vi "Initialize.vi"(8 "error in (no error)":errorcluster, 10 "Simulated Custom Devices":refnum<class "Simulated VeriStand Custom Device.lvclass">[](array[class]), 11 "Simulated VeriStand Engine in":refnum<class "Simulated VeriStand Engine.lvclass">) -> (0 "error out":errorcluster, 3 "Simulated VeriStand Engine out":refnum<class "Simulated VeriStand Engine.lvclass">)   [LabVIEW 2016, in "Simulated VeriStand Engine.lvclass"]
uses:
  Simulated VeriStand Engine.lvclass
  Simulated VeriStand Custom Device/Simulated VeriStand Custom Device.lvclass
  Simulated VeriStand Engine.lvclass/Simulated VeriStand Engine.ctl
  <vilib>/NI Veristand/Custom Device API/Data Table Ref.ctl
  Typedefs/DSF.Engine.Pointers.Control.ctl
  Source/Submodules/Memory/Source/Classes/Internal/Memory.Pointer.Internal.lvclass
  C:/Git/SourceTree/DSF/Source/Submodules/Memory/Source/Classes/Pointer/Memory.Pointer.lvclass
  Typedefs/DSF.Engine.Pointers.Status.ctl
  Source/Submodules/Memory/Source/Classes/Pointer/Memory.Pointer.lvclass/Memory.Pointer.ctl
  Source/Submodules/Memory/Source/Classes/Pointer/Memory.Pointer.Write.Safe.0D.Bool.vi
  Source/Submodules/Memory/Source/Classes/Pointer/Memory.Pointer.Write.Safe.0D.U32.vi
  Source/Submodules/Memory/Source/Classes/Pointer/Memory.Pointer.Write.Unsafe.0D.Bool.vi
  Source/Submodules/Memory/Source/Classes/Pointer/Memory.Pointer.Parameter Check.Null Pointer.vi
  Source/Submodules/Memory/Source/Classes/Pointer/Memory.Pointer.Parameter Check.Subset.vi
  Source/Submodules/Memory/Source/Classes/Pointer/Memory.Pointer.Write.Unsafe.0D.U32.vi
  Source/Submodules/Memory/Source/Classes/Pointer/Memory.Pointer.Get Address.vi
  Source/Submodules/Memory/Source/Classes/Pointer/Memory.Pointer.Errors.vi
  Source/Submodules/Memory/Source/Classes/Pointer/Memory.Pointer.Errors.Null Pointer.vi
  Source/Submodules/Memory/Source/Classes/Pointer/Memory.Pointer.Errors.Out of Bounds.vi
  Source/Submodules/Memory/Source/Classes/Pointer/Memory.Pointer.Get Size.vi
  Source/Submodules/Memory/Source/Classes/Pointer/Memory.Pointer.Errors.Create Error.vi
  Source/Submodules/Memory/Source/Submodules/SEH/Source/VIs/Static Error Handling.Source Buffer.Write.String.vi
  Source/Submodules/Memory/Source/Classes/Pointer/Memory.Pointer.Errors.Write Pointer Size.vi
  Source/Submodules/Memory/Source/Submodules/SEH/Source/VIs/Static Error Handling.Source Buffer.Write.Numeric.Scalar.Base10.vi
  Source/Submodules/Memory/Source/Submodules/SEH/Source/VIs/Static Error Handling.Source Buffer.Write.Numeric.Scalar.Base10 (U64).vi
  Source/Submodules/Memory/Source/Submodules/SEH/Source/VIs/Static Error Handling.Error Cluster Constant.vi
  Source/Submodules/Memory/Source/Submodules/SEH/Source/VIs/Static Error Handling.Error Cluster Constant (256B).vi
  Source/Submodules/Memory/Source/Submodules/SEH/Source/VIs/Static Error Handling.Parameters.Status.Set.vi
  Source/Submodules/Memory/Source/Submodules/SEH/Source/VIs/Static Error Handling.Parameters.Code.Set.vi
  Source/Submodules/Memory/Source/Submodules/SEH/Source/VIs/Static Error Handling.Parameters.VI Source.Set.vi
  Source/Submodules/Memory/Source/Constants/Memory.Constants.vi
  Source/Submodules/Memory/Source/Constants/Memory.Constants.Library Name.vi
  Source/Submodules/Memory/Source/Classes/Pointer/Memory.Pointer.Errors.Get Info.vi
  Source/Submodules/Memory/Source/Classes/Internal/Memory.Pointer.Internal.Allocate.vi
  <vilib>/NI Veristand/Custom Device API/Global Data Refs.vi
  <vilib>/NI Veristand/Custom Device API/Custom Device API.lvlib
  Source/Submodules/Memory/Source/Classes/Pointer/Memory.Pointer.lvclass
panel:
  in  "Channel Count":u32
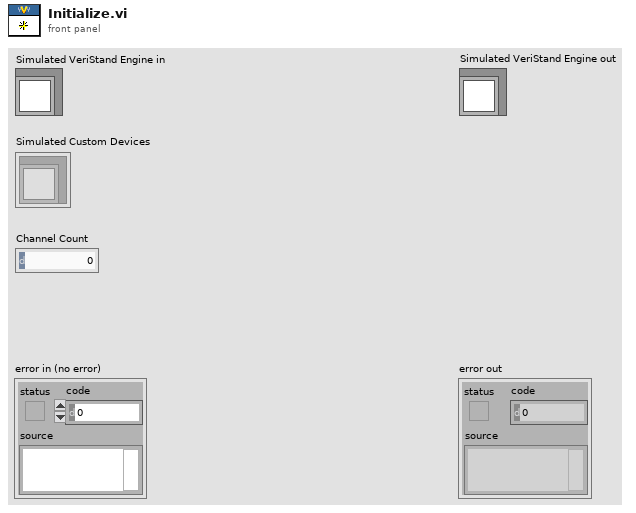
[diagram p1: front panel]
types:
  T1 = typedef "Simulated VeriStand Engine.lvclass/DSF.Engine.Pointers.Status.ctl" = cluster{"actual period":refnum<class "Memory.Pointer.Internal.lvclass">}
  T2 = typedef "Simulated VeriStand Engine.lvclass/DSF.Engine.Pointers.Control.ctl" = cluster{"stop":refnum<class "Memory.Pointer.Internal.lvclass">, "target period":refnum<class "Memory.Pointer.Internal.lvclass">}
  T3 = typedef "Custom Device API.lvlib/Data Table Ref.ctl" = cluster{"Ptr.Beg":u64, "Ptr.End":u64}
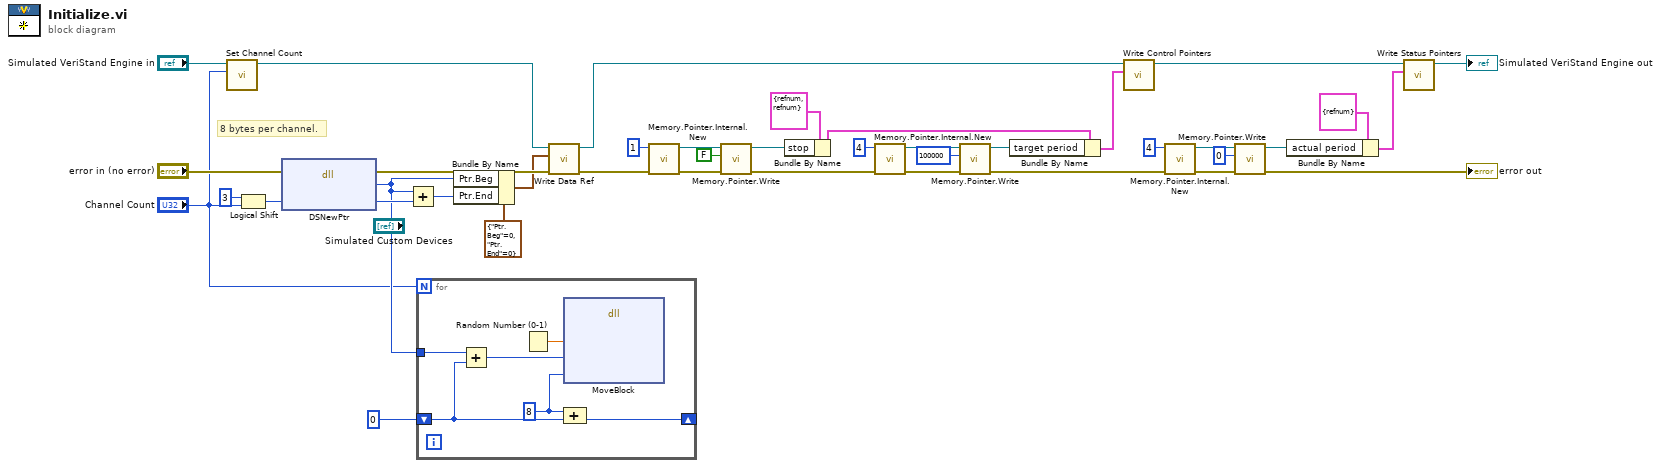
[diagram p0: block diagram]
diagram:
  # "8 bytes per channel."
  n1 = call "Set Channel Count.vi"("Channel Count"="Channel Count", "Simulated VeriStand Engine in"="Simulated VeriStand Engine in") -> ("Simulated VeriStand Engine out"=w2:refnum<class "Simulated VeriStand Engine.lvclass">)  [unwired: 8 in, 1 out]
  n2 = Logical Shift(y=i16 3, x="Channel Count") -> (x << y=w39:u32)
  n3 = dll-call lib="LabVIEW" fn="DSNewPtr"(error in="error in (no error)", "size"=w39) -> (error out=w5:errorcluster, "pointer"=w8:u64, "size"=w36:u32)  [unwired: 2 in, 1 out]
  n4 = Add(x=w8, y=w36) -> (x+y=w37:u64)
  n5 = for {
    N: "Channel Count" -> [_]
    tunnel: w8 -> [w45]
    shift-right: [w44] -> _
    shift-left: u64 0 -> [w43]
    w41 = u64 8
    n6 = Add(x=w45, y=w43) -> (x+y=w42:u64)
    n7 = Random Number (0-1)() -> (number: 0 to 1=w46:dbl)
    n8 = dll-call lib="LabVIEW" fn="MoveBlock"("src"=w46, "dst"=w42, "size"=w41) -> ()  [unwired: 7 in, 2 out]
    n9 = Compound Arithmetic op=ADD(w41, w43) -> (w44:u64)
  }
  n10 = Bundle By Name(cluster=T3 {"Ptr.Beg"=0, "Ptr.End"=0} ("Data Ref"), "Ptr.Beg"=w8, "Ptr.End"=w37) -> (w3:T3)
  n11 = call "Write Data Ref.vi"("error in (no error)"=w5, "Data Table Ref"=w3, "Simulated VeriStand Engine in"=w2) -> ("error out"=w4:errorcluster, "Simulated VeriStand Engine out"=w1:refnum<class "Simulated VeriStand Engine.lvclass">)  [unwired: 7 in]
  n12 = call "Memory.Pointer.Internal.New.vi"("error in (no error)"=w4, "size"=u64 1) -> ("error out"=w22:errorcluster, "pointer"=w23:refnum<class "Memory.Pointer.Internal.lvclass">)  [unwired: 8 in]
  n13 = call-poly "Memory.Pointer.Write.vi"("error in (no error)"=w22, "value"=FALSE, "pointer in"=w23) -> ("error out"=w16:errorcluster, "pointer out"=w20:refnum<class "Memory.Pointer.Internal.lvclass">)  [unwired: 5 in, 2 out]
  n14 = Bundle By Name(cluster=T2 {"stop"=refnum, "target period"=refnum} ("Control Pointers"), "stop"=w20) -> (w29:T2)
  n15 = call "Memory.Pointer.Internal.New.vi"("error in (no error)"=w16, "size"=u64 4) -> ("error out"=w17:errorcluster, "pointer"=w19:refnum<class "Memory.Pointer.Internal.lvclass">)  [unwired: 8 in]
  n16 = call-poly "Memory.Pointer.Write.vi"("error in (no error)"=w17, "value"=u32 100000, "pointer in"=w19) -> ("error out"=w11:errorcluster, "pointer out"=w10:refnum<class "Memory.Pointer.Internal.lvclass">)  [unwired: 5 in, 2 out]
  n17 = Bundle By Name(cluster=w29, "target period"=w10) -> (w28:T2)
  n18 = call "Write Control Pointers.vi"("Control Pointers"=w28, "Simulated VeriStand Engine in"=w1) -> ("Simulated VeriStand Engine out"=w33:refnum<class "Simulated VeriStand Engine.lvclass">)  [unwired: 8 in, 1 out]
  n19 = call "Memory.Pointer.Internal.New.vi"("error in (no error)"=w11, "size"=u64 4) -> ("error out"=w14:errorcluster, "pointer"=w15:refnum<class "Memory.Pointer.Internal.lvclass">)  [unwired: 8 in]
  n20 = call-poly "Memory.Pointer.Write.vi"("error in (no error)"=w14, "value"=u32 0, "pointer in"=w15) -> ("error out"=→"error out":errorcluster, "pointer out"=w13:refnum<class "Memory.Pointer.Internal.lvclass">)  [unwired: 5 in, 2 out]
  n21 = Bundle By Name(cluster=T1 {"actual period"=refnum} ("Status Pointers"), "actual period"=w13) -> (w25:T1)
  n22 = call "Write Status Pointers.vi"("Status Pointers"=w25, "Simulated VeriStand Engine in"=w33) -> ("Simulated VeriStand Engine out"=→"Simulated VeriStand Engine out":refnum<class "Simulated VeriStand Engine.lvclass">)  [unwired: 8 in, 1 out]
